vi "test-trapezoid-profile-top-speed.vi"() -> (3 "Test Passed":bool)   [LabVIEW 2019]
uses:
  <vilib>/Rock Robotics/WPI/ThirdParty/JAS_Junk/TrajLib/TRAPEZOID_PROFILE_STATE.ctl
  <vilib>/Rock Robotics/WPI/ThirdParty/JAS_Junk/TrajLib/TRAPEZOID_PROFILE.ctl
  <vilib>/Rock Robotics/WPI/ThirdParty/JAS_Junk/TrajLib/TRAPEZOID_PROFILE_CONSTRAINT.ctl
  <vilib>/Rock Robotics/WPI/ThirdParty/JAS_Junk/TrajLib/TrapProfile_ShouldFlipAcceleration.vi
  <vilib>/Rock Robotics/WPI/ThirdParty/JAS_Junk/TrajLib/TrapProfile_Direct.vi
  <vilib>/Rock Robotics/SystemInterfaces/NetworkCommunication/NetComm_UsageReport_report.vi
  <vilib>/Rock Robotics/WPI/ThirdParty/JAS_Junk/TrajLib/Util_LibraryGlobals.vi
  <vilib>/Rock Robotics/WPI/ThirdParty/JAS_Junk/TrajLib/Trajectory_Library.lvlib
panel:
  out "Goal":T1 {"Velocity" format="%16_6e"; "Position" format="%16_6e"}
  out "ApproxEquals 2":bool
  out "ApproxEquals":bool
  out "Equal":bool
  out "State 2":T1 {"Velocity" format="%16_6e"; "Position" format="%16_6e"}
  out "Waveform Chart 2":T2(graph)
  out "TRAPEZOID_PROFILE 2":T3 {"Goal"."Velocity" format="%16_6e"; "Goal"."Position" format="%16_6e"; "Initial"."Velocity" format="%16_6e"; "Initial"."Position" format="%16_6e"; "Constraints"."MaxAcceleration" format="%16_6e"; "Constraints"."MaxVelocity" format="%16_6e"; "EndDecel" format="%16_6e"; "EndFullSpeed" format="%16_6e"; "EndAccel" format="%16_6e"}
  out "TRAPEZOID_PROFILE":T3 {"Goal"."Velocity" format="%16_6e"; "Goal"."Position" format="%16_6e"; "Initial"."Velocity" format="%16_6e"; "Initial"."Position" format="%16_6e"; "Constraints"."MaxAcceleration" format="%16_6e"; "Constraints"."MaxVelocity" format="%16_6e"; "EndDecel" format="%16_6e"; "EndFullSpeed" format="%16_6e"; "EndAccel" format="%16_6e"}
  out "State":T1 {"Velocity" format="%16_6e"; "Position" format="%16_6e"}
  out "Waveform Chart":T2(graph)
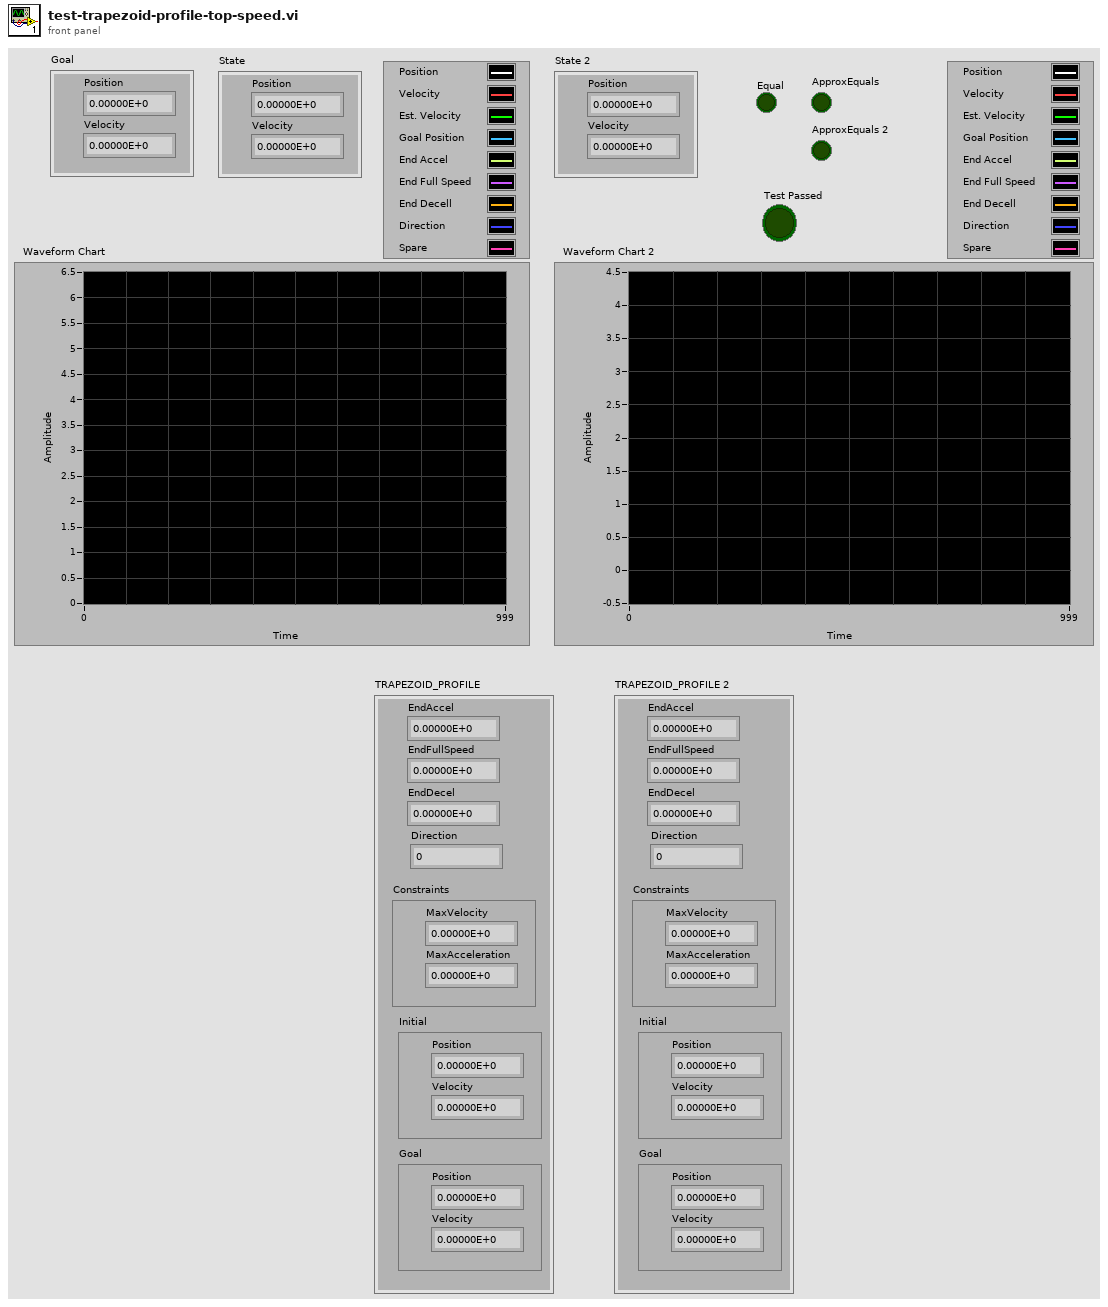
[diagram p1: front panel]
types:
  T1 = typedef "Trajectory_Library.lvlib/TRAPEZOID_PROFILE_STATE.ctl" = cluster{"Position":dbl, "Velocity":dbl}
  T2 = cluster{"Position":dbl, "Velocity":dbl, dbl, "Position":dbl, "EndAccel":dbl, "EndFullSpeed":dbl, "EndDecel":dbl, "Direction":i32, "Position":dbl}
  T3 = typedef "Trajectory_Library.lvlib/TRAPEZOID_PROFILE.ctl" = cluster{"EndAccel":dbl, "EndFullSpeed":dbl, "EndDecel":dbl, "Direction":i32, "Constraints":T4, "Initial":T1, "Goal":T1}
  T4 = typedef "Trajectory_Library.lvlib/TRAPEZOID_PROFILE_CONSTRAINT.ctl" = cluster{"MaxVelocity":dbl, "MaxAcceleration":dbl}
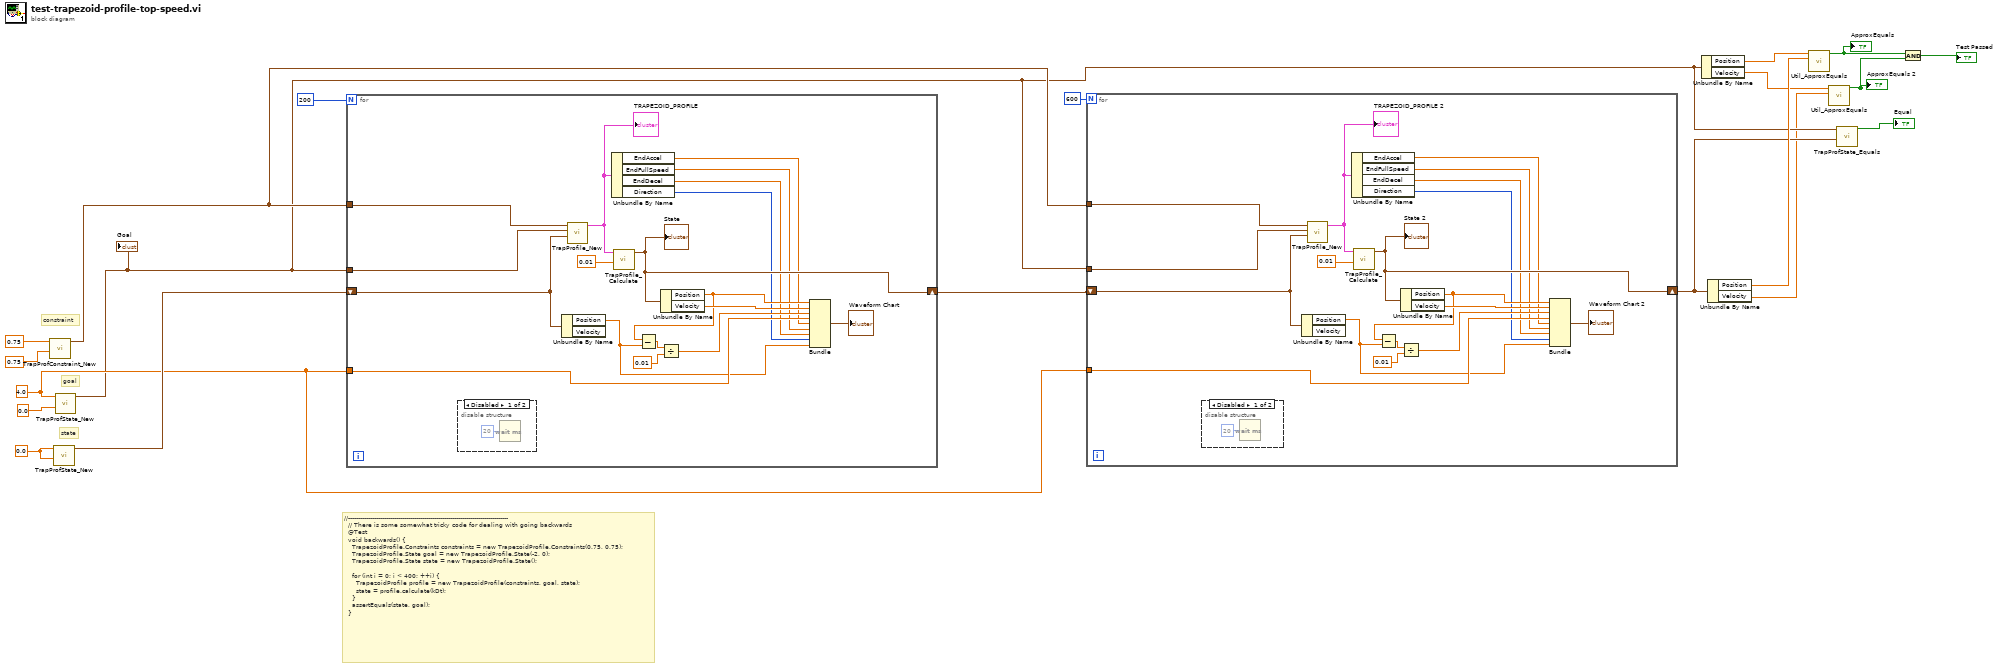
[diagram p0: block diagram]
diagram:
  w16 = 0.0 ("Position")
  w11 = 4.0 ("Position")
  # "state"
  # "//--------------------------------------------------------------------------------\n  // There is some somewhat tricky code for dealing with going backwards\n  @Test\n  void backwards() {\n    TrapezoidProfile.Constraints constraints = new TrapezoidProfile.Constraints(0.75, 0.75);\n    TrapezoidProfile.State goal = new TrapezoidProfile.State(-2, 0);\n    TrapezoidProfile.State state = new TrapezoidProfile.State();\n\n    for (int i = 0; i < 400; ++i) {\n      TrapezoidProfile profile = new TrapezoidProfile(constraints, goal, state);\n      state = profile.calculate(kDt);\n    }\n    assertEquals(state, goal);\n  }"
  # "goal"
  # "constraint"
  n1 = call <vilib>:"TrapProfConstraint_New.vi"("Max Accel"=0.75, "Max Speed (M/S)"=0.75) -> ("TRAPEZOID_PROFILE_CONSTRAINT"=w12:T4)  [unwired: 9 in]
  n2 = call <vilib>:"TrapProfState_New.vi"("Velocity"=w16, "Position"=w16) -> ("TRAPEZOID_PROFILE_STATE"=w15:T1)  [unwired: 9 in]
  n3 = call <vilib>:"TrapProfState_New.vi"("Velocity"=0.0, "Position"=w11) -> ("TRAPEZOID_PROFILE_STATE"=w7:T1)  [unwired: 9 in]
  "Goal" <- w7
  n4 = for {
    N: 200 -> [_]
    shift-right: [w29] -> w13
    shift-left: w15 -> [w34]
    tunnel: w7 -> [w36]
    tunnel: w11 -> [w28]
    tunnel: w12 -> [w21]
    n5 = disable-structure shown="Disabled" {
      frame Disabled {
        n6 = Wait (ms)(milliseconds to wait=u32 20) -> ()  [unwired: 1 out]
      }
      frame Enabled {
      }
    }
    n7 = Unbundle By Name(w34) -> ("Position"=w22:dbl)  [unwired: 1 out]
    n8 = call <vilib>:"TrapProfile_New.vi"("Initial"=w34, "Goal"=w36, "Constraints"=w21) -> ("TRAPEZOID_PROFILE"=w27:T3)  [unwired: 8 in]
    "TRAPEZOID_PROFILE" <- w27
    n9 = Unbundle By Name(w27) -> ("EndAccel"=w26:dbl, "EndFullSpeed"=w25:dbl, "EndDecel"=w24:dbl, "Direction"=w23:i32)
    n10 = call <vilib>:"TrapProfile_Calculate.vi"("Time"=0.01, "TRAPEZOID_PROFILE"=w27) -> ("State"=w29:T1)  [unwired: 9 in]
    "State" <- w29
    n11 = Unbundle By Name(w29) -> ("Position"=w33:dbl, "Velocity"=w37:dbl)
    n12 = Subtract(x=w33, y=w22) -> (x-y=w32:dbl)
    n13 = Divide(x=w32, y=0.01) -> (x/y=w30:dbl)
    n14 = Bundle("Position"=w33, "Velocity"=w37, w30, "Position"=w28, "EndAccel"=w26, "EndFullSpeed"=w25, "EndDecel"=w24, "Direction"=w23, "Position"=w22) -> (→"Waveform Chart":T2)  [unwired: 1 in]
  }
  n15 = for {
    N: 600 -> [_]
    shift-right: [w48] -> w6
    shift-left: w13 -> [w53]
    tunnel: w7 -> [w55]
    tunnel: w11 -> [w47]
    tunnel: w12 -> [w40]
    n16 = disable-structure shown="Disabled" {
      frame Disabled {
        n17 = Wait (ms)(milliseconds to wait=u32 20) -> ()  [unwired: 1 out]
      }
      frame Enabled {
      }
    }
    n18 = Unbundle By Name(w53) -> ("Position"=w41:dbl)  [unwired: 1 out]
    n19 = call <vilib>:"TrapProfile_New.vi"("Initial"=w53, "Goal"=w55, "Constraints"=w40) -> ("TRAPEZOID_PROFILE"=w46:T3)  [unwired: 8 in]
    "TRAPEZOID_PROFILE 2" <- w46
    n20 = Unbundle By Name(w46) -> ("EndAccel"=w45:dbl, "EndFullSpeed"=w44:dbl, "EndDecel"=w43:dbl, "Direction"=w42:i32)
    n21 = call <vilib>:"TrapProfile_Calculate.vi"("Time"=0.01, "TRAPEZOID_PROFILE"=w46) -> ("State"=w48:T1)  [unwired: 9 in]
    "State 2" <- w48
    n22 = Unbundle By Name(w48) -> ("Position"=w52:dbl, "Velocity"=w56:dbl)
    n23 = Subtract(x=w52, y=w41) -> (x-y=w51:dbl)
    n24 = Divide(x=w51, y=0.01) -> (x/y=w49:dbl)
    n25 = Bundle("Position"=w52, "Velocity"=w56, w49, "Position"=w47, "EndAccel"=w45, "EndFullSpeed"=w44, "EndDecel"=w43, "Direction"=w42, "Position"=w41) -> (→"Waveform Chart 2":T2)  [unwired: 1 in]
  }
  n26 = Unbundle By Name(w7) -> ("Position"=w10:dbl, "Velocity"=w8:dbl)
  n27 = Unbundle By Name(w6) -> ("Position"=w9:dbl, "Velocity"=w4:dbl)
  n28 = call <vilib>:"Util_ApproxEquals.vi"("Value 2"=w9, "Value 1"=w10) -> ("ApproxEquals"=w2:bool)  [unwired: 9 in]
  "ApproxEquals" <- w2
  n29 = call <vilib>:"Util_ApproxEquals.vi"("Value 2"=w4, "Value 1"=w8) -> ("ApproxEquals"=w1:bool)  [unwired: 9 in]
  "ApproxEquals 2" <- w1
  n30 = call <vilib>:"TrapProfState_Equals.vi"("TRAPEZOID_PROFILE_STATE 2"=w6, "TRAPEZOID_PROFILE_STATE"=w7) -> ("Equal"=→"Equal":bool)  [unwired: 9 in]
  n31 = And(x=w2, y=w1) -> (x .and. y?=→"Test Passed":bool)
